vi "Test Suite from LVLib.vi"(8 "error in (no error)":errorcluster, 11 "Test Case In":refnum<class "LUnit Test Suite Tests.lvclass">) -> (0 "error out":errorcluster, 3 "Test Case Out":refnum<class "LUnit Test Suite Tests.lvclass">)   [LabVIEW 2020, in "LUnit Test Suite Tests.lvclass"]
uses:
  LUnit Test Suite Tests.lvclass
  source/API/LUnit Test Suite/LUnit Test Suite.lvclass
  C:/git/astemes-lunit/source/Core/Runnable/Runnable.lvclass
  LUnit Test Suite Tests.lvclass/LUnit Test Suite Tests.ctl
  source/API/Test Suite Factory/Test Suite Factory.lvclass
  source/Core/Runnable/Runnable.lvclass
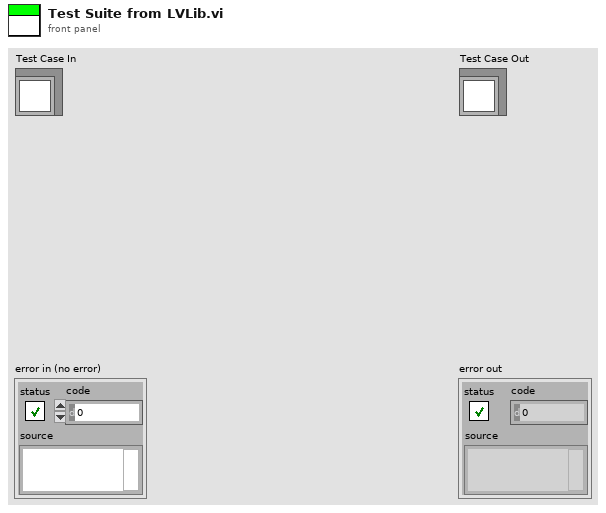
[diagram p1: front panel]
types:
  T1 = typedef "Result.lvlib/Result.ctl" = cluster{"Name":string, "Message":string, "Description":string, "Status":T2, "Result Type":T3, "Execution Time":dbl}
  T2 = typedef "Result.lvlib/Status.ctl" = enum16{"", "Passed", "Failed", "Error", "Skipped", "Setup Error", "Broken", "Teardown Error"}
  T3 = typedef "Result.lvlib/Type.ctl" = enum16{"Test Case", "Test Suite", "Test Run", "Pass", "Fail", "Skip", "Pass if", "Fail if", "Pass if Error", "Fail if Error", "Pass if Equal", "Fail if Equal"}
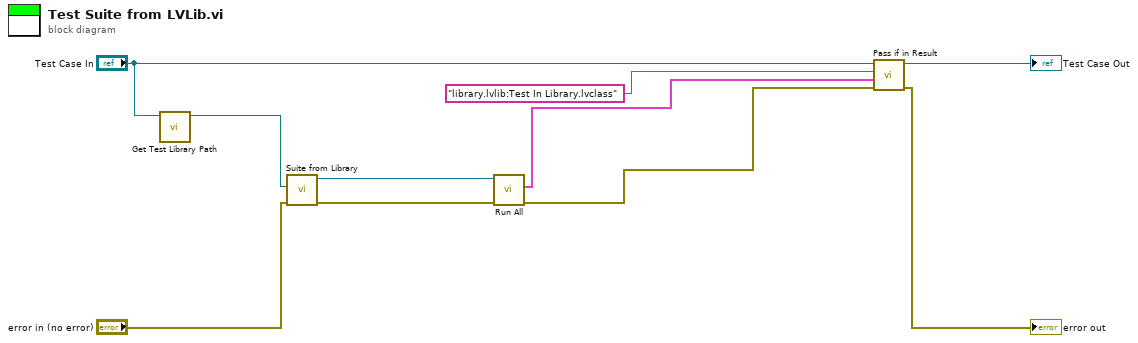
[diagram p0: block diagram]
diagram:
  n1 = call "Get Test Library Path.vi"("LUnit Test Suite Tests in"="Test Case In") -> ("lvlib path"=w7:path)  [unwired: 9 in, 1 out]
  n2 = call "Suite from Library.vi"("error in (no error)"="error in (no error)", "Library Path"=w7) -> ("error out"=w6:errorcluster, "LUnit Test Suite Out"=w2:refnum<class "LUnit Test Suite.lvclass">)  [unwired: 8 in]
  n3 = call "Run All.vi"("error in (no error)"=w6, "Runnable In"=w2) -> ("error out"=w5:errorcluster, "Results"=w1:T1[])  [unwired: 8 in]
  n4 = call "Pass if in Result.vi"("error in (no error)"=w5, "Results"=w1, "Method Name"="library.lvlib:Test In Library.lvclass" ("class name"), "LUnit Test Suite Tests in"="Test Case In") -> ("error out"=→"error out":errorcluster, "LUnit Test Suite Tests out"=→"Test Case Out":refnum<class "LUnit Test Suite Tests.lvclass">)  [unwired: 6 in]
